vi "To Variant.vi"(8 "error in":errorcluster, 11 "Boolean in":refnum<class "Double.lvclass">) -> (0 "error out":errorcluster, 3 "Variant":variant)   [LabVIEW 2020, in "Double.lvclass"]
uses:
  <vilib>/gpm_packages/@cs/data-type-serializer/source/Double/Double.lvclass
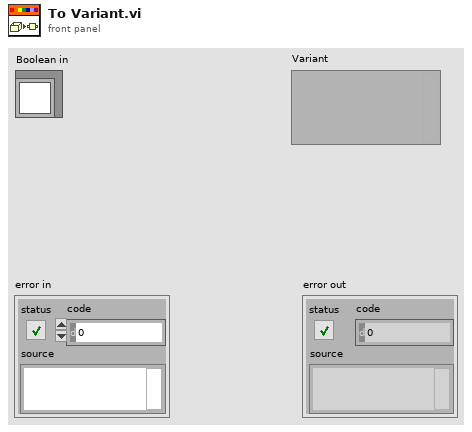
[diagram p1: front panel]
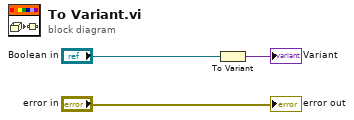
[diagram p0: block diagram]
diagram:
  n1 = To Variant(anything="Boolean in") -> (Variant=→"Variant":variant)
  "error out" <- "error in"
